vi "SubVIConcept.vi"() -> ()   [LabVIEW 2019]
panel:
  out "EngineTempF":dbl
  in  "EngineTempC":dbl
  out "BoilerTempF":dbl
  in  "BoilderTempC":dbl
  out "TempF":dbl
  in  "TempC":dbl
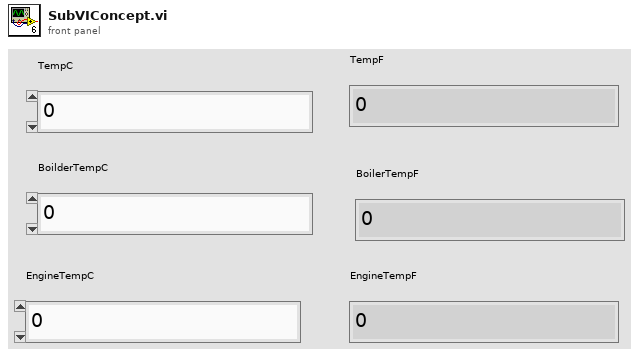
[diagram p1: front panel]
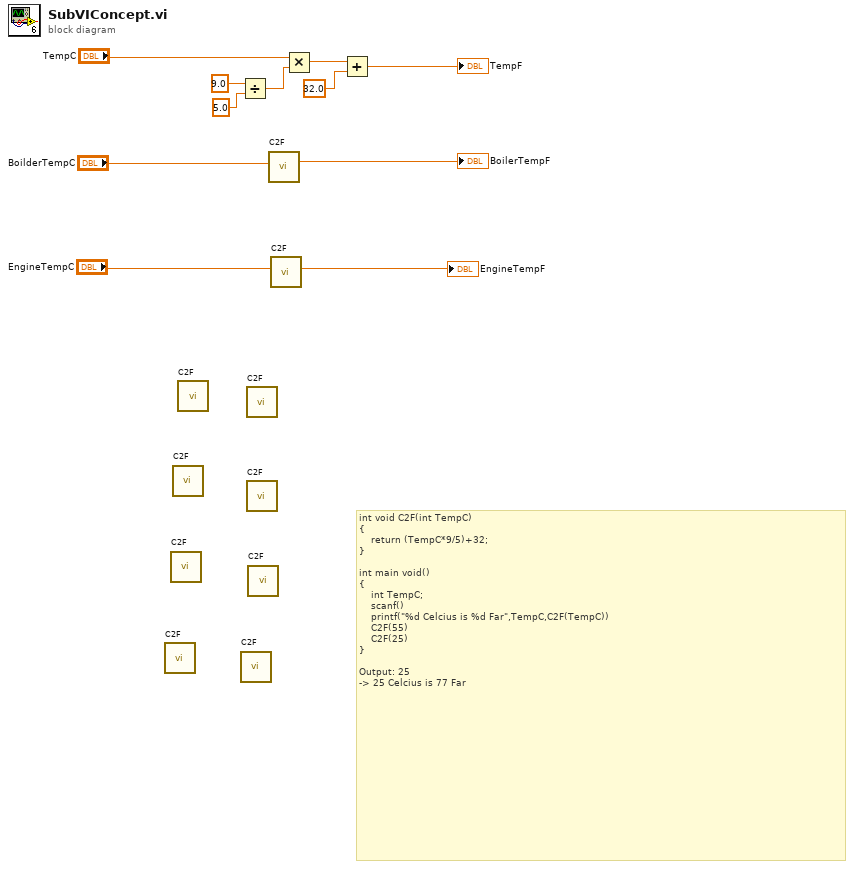
[diagram p0: block diagram]
diagram:
  # "int void C2F(int TempC)\n{\n    return (TempC*9/5)+32;\n}\n\nint main void()\n{\n    int TempC;\n    scanf()\n    printf(\"%d Celcius is %d Far\",TempC,C2F(TempC))\n    C2F(55)\n    C2F(25)\n}\n\nOutput: 25\n-> 25 Celcius is 77 Far"
  n1 = call "C2F.vi"() -> ()  [unwired: 11 in, 1 out]
  n2 = call "C2F.vi"() -> ()  [unwired: 11 in, 1 out]
  n3 = call "C2F.vi"() -> ()  [unwired: 11 in, 1 out]
  n4 = call "C2F.vi"() -> ()  [unwired: 11 in, 1 out]
  n5 = Divide(x=9.0, y=5.0 ("x")) -> (x/y=w10:dbl)
  n6 = call "C2F.vi"() -> ()  [unwired: 11 in, 1 out]
  n7 = call "C2F.vi"() -> ()  [unwired: 11 in, 1 out]
  n8 = call "C2F.vi"() -> ()  [unwired: 11 in, 1 out]
  n9 = call "C2F.vi"() -> ()  [unwired: 11 in, 1 out]
  n10 = call "C2F.vi"("TempC"="BoilderTempC") -> ("TempF"=→"BoilerTempF":dbl)  [unwired: 10 in]
  n11 = call "C2F.vi"("TempC"="EngineTempC") -> ("TempF"=→"EngineTempF":dbl)  [unwired: 10 in]
  n12 = Multiply(x="TempC", y=w10) -> (x*y=w7:dbl)
  n13 = Add(x=w7, y=32.0) -> (x+y=→"TempF":dbl)
